vi "Begin.vi"(11 "Image Size":T1=enum."160x120") -> (0 "error out":errorcluster)   [LabVIEW 2013]
doc: "Called before other user functions, this VI is expected to open initial I/O refnums, load in file data, and do all program initialization. Notice that the <B>error out</B> terminal is simply used for data flow. Wiring it to other structures or subVIs ensures that this VI runs first."
uses:
  <vilib>/Rock Robotics/WPI/Camera/WPI_CameraImageSize.ctl
  <vilib>/Rock Robotics/WPI/Camera/WPI_CameraWhite Balance Values.ctl
  <vilib>/Rock Robotics/WPI/Camera/WPI_CameraExposure Values.ctl
  <vilib>/Rock Robotics/WPI/Camera/WPI_CameraFrameRate.ctl
  <vilib>/Rock Robotics/WPI/DriverStation/WPI_DriverStationRobotMode2.ctl
  <vilib>/Rock Robotics/WPI/Joystick/WPI_JoystickDeviceEnum.ctl
  <vilib>/Rock Robotics/SystemInterfaces/DIO/FPGA_DIOPWMChannel.ctl
  <vilib>/Rock Robotics/SystemInterfaces/DIO/FPGA_DIOChannel.ctl
  <vilib>/Rock Robotics/WPI/Solenoid/WPI_SolenoidChannel.ctl
  <vilib>/Rock Robotics/SystemInterfaces/DIO/FPGA_DIORelayChannel.ctl
  <vilib>/Rock Robotics/WPI/SafetyOutput/WPI_SafetyOutputConfigMenu.ctl
  <vilib>/Rock Robotics/SystemInterfaces/Typedef/FPGA_TypedefSolenoidModule.ctl
  <vilib>/Rock Robotics/WPI/Encoder/WPI_EncoderType.ctl
  <vilib>/Rock Robotics/WPI/Relay/WPI_RelayValue.ctl
  <vilib>/Rock Robotics/SystemInterfaces/Typedef/FPGA_TypedefDigitalModule.ctl
  Robot Global Data.vi
  <vilib>/Rock Robotics/WPI/MotorControl/WPI_MotorControlOpen Talon.vi
  <vilib>/Rock Robotics/WPI/Counter/WPI_CounterDigitalInputToDigitalSource.vi
  <vilib>/Rock Robotics/WPI/RobotDrive/WPI_RobotDriveOpen2MotorWithTalon.vi
  <vilib>/Rock Robotics/WPI/Solenoid/WPI_SolenoidOpenDouble.vi
  <vilib>/Rock Robotics/WPI/Compressor/WPI_CompressorGetSetRefNum.vi
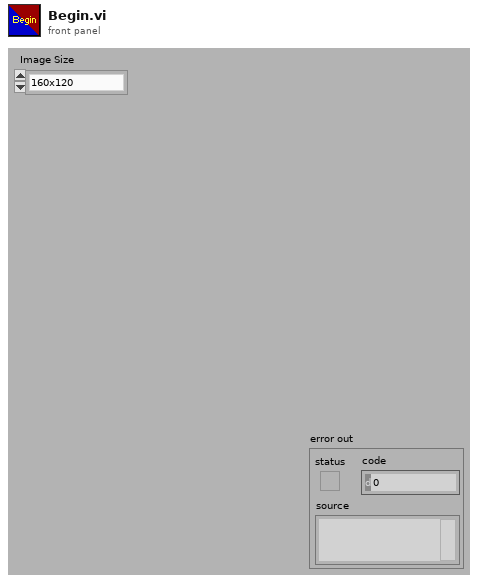
[diagram p1: front panel]
types:
  T1 = typedef "WPI_CameraImageSize.ctl" = enum16{"640x480", "320x240", "160x120"}
  T2 = typedef "FPGA_DIOPWMChannel.ctl" = enum8{"PWM 1", "PWM 2", "PWM 3", "PWM 4", "PWM 5", "PWM 6", "PWM 7", "PWM 8", "PWM 9", "PWM 10", "Invalid"}
  T3 = typedef "FPGA_TypedefDigitalModule.ctl" = enum16{"Digital Module 1", "Digital Module 2"}
  T4 = typedef "WPI_RelayValue.ctl" = enum16{"Off", "On", "Forward", "Reverse"}
  T5 = typedef "FPGA_DIORelayChannel.ctl" = enum8{"Relay 1", "Relay 2", "Relay 3", "Relay 4", "Relay 5", "Relay 6", "Relay 7", "Relay 8", "Invalid"}
  T6 = typedef "WPI_EncoderType.ctl" = enum16{"1x", "2x", "4x"}
  T7 = typedef "FPGA_DIOChannel.ctl" = enum8{"DIO 1", "DIO 2", "DIO 3", "DIO 4", "DIO 5", "DIO 6", "DIO 7", "DIO 8", "DIO 9", "DIO 10", "DIO 11", "DIO 12", "DIO 13", "DIO 14", "Invalid"}
  T8 = typedef "FPGA_TypedefSolenoidModule.ctl" = enum16{"Solenoid Module 1", "Solenoid Module 2"}
  T9 = typedef "WPI_SafetyOutputConfigMenu.ctl" = enum16{"Enable", "Disable"}
  T10 = typedef "WPI_SolenoidChannel.ctl" = enum8{"Solenoid 1", "Solenoid 2", "Solenoid 3", "Solenoid 4", "Solenoid 5", "Solenoid 6", "Solenoid 7", "Solenoid 8", "Invalid"}
  T11 = typedef "WPI_JoystickDeviceEnum.ctl" = enum16{"USB 1", "USB 2", "USB 3", "USB 4", "Kinect 1", "Kinect 2"}
  T12 = typedef "WPI_DriverStationRobotMode2.ctl" = enum16{"Autonomous Disabled", "Autonomous Enabled", "Teleop Disabled", "Teleop Enabled", "Timeout", "Finish", "Test Disabled", "Test Enabled"}
  T13 = typedef "WPI_CameraFrameRate.ctl" = u32
  T14 = typedef "WPI_CameraExposure Values.ctl" = enum16{"Auto", "Flicker-free 50 Hz", "Flicker-free 60 Hz", "Hold current"}
  T15 = typedef "WPI_CameraWhite Balance Values.ctl" = enum16{"Auto", "Fixed indoor", "Fixed outdoor 1", "Fixed outdoor 2", "Fixed fluorescent 1", "Fixed fluorescent 2", "Hold current"}
  T16 = typedef "WPI_JoystickDevRef.ctl" = cluster{"Device":T11}
  T17 = typedef "WPI_RobotDriveDevRef.ctl" = cluster{"DevStatus":errorcluster, "Motors[]":T18[], "Square Inputs":bool, "Max Output":dbl, "Isochronous":bool}
  T18 = typedef "WPI_MotorControlDeviceRef.ctl" = cluster{"DeviceStatus":errorcluster, "Type":enum16{"PWM", "CAN"}, "PWM":cluster{"Digital Module":T3, "PWM Channel":T2, "DeadBand":T19}, "CAN":cluster{"Device Number":u8, "Control Mode":T20, "Semaphore":T21, "Max Vout":dbl}, "Invert":bool, "TransformRef":T22, "InvTransformRef":T22}
  T19 = typedef "WPI_PWMDeadband.ctl" = cluster{"Name":string, "maxPositivePwm":i32, "minPositivePwm":i32, "centerPwm":i32, "maxNegativePwm":i32, "minNegativePwm":i32, "angularRange":u16}
  T20 = typedef "WPI_CANJaguar_ControlMode.ctl" = enum8{"Percent VBus", "Current", "Speed", "Position", "Voltage"}
  T21 = typedef "Semaphore RefNum" = refnum<k1>
  T22 = typedef "WPI_PWMTransform_ConPane.ctl" = refnum<vi>
  T23 = typedef "WPI_CameraDevRef.ctl" = cluster{"Camera Address":string, "CameraStatus":errorcluster, "Acquire Image Notifier":refnum<notifier>}
  T24 = typedef "WPI_DigitalInputDevRef.ctl" = cluster{"DevStatus":errorcluster, "DIO Channel":T7, "Digital Module":T3}
  T25 = typedef "WPI_CompressorDevRef.ctl" = cluster{"DevStatus":errorcluster, "DigitalInputDevRef":T24, "RelayDevRef":T26}
  T26 = typedef "WPI_RelayDevRef.ctl" = cluster{"DevStatus":errorcluster, "Relay Channel":T5, "Digital Module":T3, "Relay Direction":T27}
  T27 = typedef "WPI_RelayDirection.ctl" = enum16{"Both directions", "Forward only", "Reverse only"}
  T28 = typedef "FPGA_CounterEncoderSourceConvertionLVSourceType.ctl" = cluster{"DevStatus":errorcluster, "AnalogTriggerMode?":bool, "DigitalMode":cluster{"Digital Module":T3, "DIO Channel":T29}, "AnalogTriggerMode":cluster{"AnalogTriggerIndex":T30, "OutputType":T31}}
  T29 = typedef "FPGA_DIODigitalSourceChannel.ctl" = enum8{"DIO 1", "DIO 2", "DIO 3", "DIO 4", "DIO 5", "DIO 6", "DIO 7", "DIO 8", "DIO 9", "DIO 10", "DIO 11", "DIO 12", "DIO 13", "DIO 14", "Disabled"}
  T30 = typedef "FPGA_AnalogTriggerIndex.ctl" = enum8{"Trig 0", "Trig 1", "Trig 2", "Trig 3", "Trig 4", "Trig 5", "Trig 6", "Trig 7", "Invalid"}
  T31 = typedef "FPGA_AnalogTriggerOutType.ctl" = enum16{"InWindow", "TriggerState", "Rising", "Falling"}
  T32 = typedef "WPI_EncoderDevRef.ctl" = cluster{"DevStatus":errorcluster, "EncoderIndex":T33, "CounterIndex":T34, "DistancePerCount":dbl, "Decoding Type":T6}
  T33 = typedef "FPGA_EncoderIdx.ctl" = enum8{"Enc 0", "Enc 1", "Enc 2", "Enc 3", "Invalid"}
  T34 = typedef "FPGA_CounterCtrSystemIndex.ctl" = enum8{"Ctr 0", "Ctr 1", "Ctr 2", "Ctr 3", "Ctr 4", "Ctr 5", "Ctr 6", "Ctr 7", "Invalid"}
  T35 = typedef "WPI_SolenoidDevRef.ctl" = cluster{"DevStatus":errorcluster, "Solenoid Module":T8, "Forward Solenoid Channel":T10, "Reverse Solenoid Channel":T10}
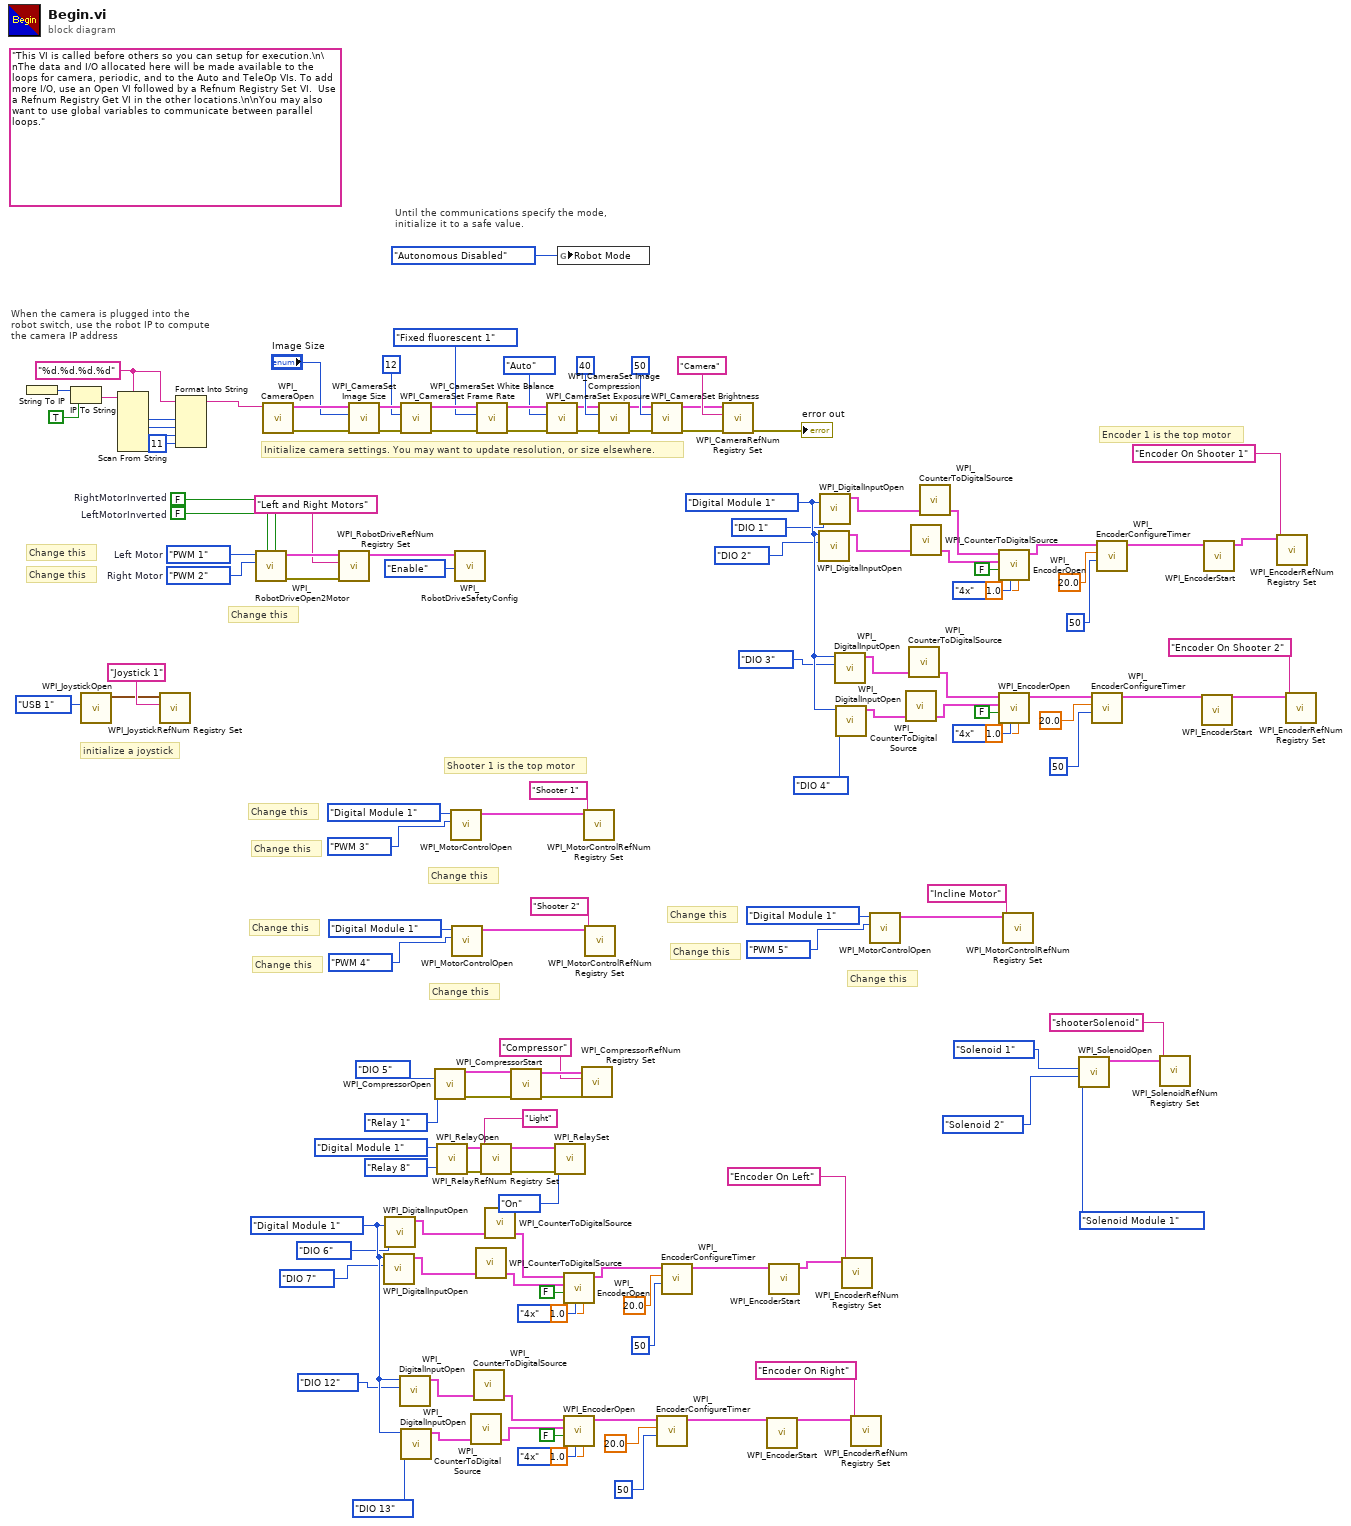
[diagram p0: block diagram]
diagram:
  w43 = FPGA_TypedefDigitalModule."Digital Module 1" ("Digital Module (Module 1)")
  w49 = FPGA_DIOPWMChannel."PWM 2"  # Right Motor
  w50 = FPGA_DIOPWMChannel."PWM 1"  # Left Motor
  w54 = FALSE  # LeftMotorInverted
  w55 = FALSE  # RightMotorInverted
  w96 = FPGA_TypedefDigitalModule."Digital Module 1" ("Digital Module (Module 1)")
  w111 = "%d.%d.%d.%d" ("format string")
  (unwired) "This VI is called before others so you can setup for execution.\n\nThe data and I/O allocated here will be made available to the loops for camera, periodic, and to the Auto and TeleOp VIs. To add more I/O, use an Open VI followed by a Refnum Registry Set VI.  Use a Refnum Registry Get VI in the other locations.\n\nYou may also want to use global variables to communicate between parallel loops."
  # "Change this"
  # "Change this"
  # "Change this"
  # "Shooter 1 is the top motor"
  # "Encoder 1 is the top motor"
  # "Change this"
  # "Change this"
  # "Change this"
  # "Change this"
  # "Change this"
  # "Change this"
  # "Change this"
  # "Change this"
  # "Change this"
  # "initialize a joystick"
  # "Until the communications specify the mode,\ninitialize it to a safe value."
  # "When the camera is plugged into the\nrobot switch, use the robot IP to compute\nthe camera IP address"
  # "Initialize camera settings. You may want to update resolution, or size elsewhere."
  n1 = String To IP() -> (0:w117:u32)  [unwired: 1 in]
  n2 = IP To String(1:TRUE ("dot notation? (F)"), 2:w117) -> (0:w115:string)
  n3 = call <vilib>:"WPI_JoystickOpen.vi"("JoystickDevice"=WPI_JoystickDeviceEnum."USB 1") -> ("JoystickDevRef"=w107:T16)  [unwired: 10 in]
  n4 = Scan From String(format string=w111, input string=w115) -> (output 1=w114:i32, output 2=w113:i32, output 3=w112:i32)  [unwired: 7 in, 3 out]
  n5 = call <vilib>:"WPI_JoystickRefNum Registry Set.vi"("refnum name"="Joystick 1", "JoystickDevRef"=w107) -> ()  [unwired: 8 in, 2 out]
  n6 = Format Into String(format string=w111, w114, w113, w112, 11 ("input 4")) -> (resulting string=w109:string)  [unwired: 2 in, 1 out]
  n7 = call-poly <vilib>:"WPI_RobotDriveOpen2Motor.vi"("Right Motor Inverted"=w55, "Left Motor Inverted"=w54, "Right Motor"=w49, "Left Motor"=w50) -> ("error out"=w51:errorcluster, "RobotDriveDevRef"=w53:T17)  [unwired: 1 in, 5 out]
  n8 = call <vilib>:"WPI_CameraOpen.vi"("Camera Address"=w109) -> ("error out"=w129:errorcluster, "CameraDevRef"=w130:T23)  [unwired: 1 in, 8 out]
  n9 = call <vilib>:"WPI_RobotDriveRefNum Registry Set.vi"("error in (no error)"=w51, "refnum name"="Left and Right Motors", "RobotDriveDevRef"=w53) -> ("RobotDriveDevRef"=w48:T17)  [unwired: 8 out]
  n10 = call <vilib>:"WPI_CameraSet Image Size.vi"("error in (no error)"=w129, "Image Size"="Image Size", "CameraDevRef"=w130) -> ("error out"=w128:errorcluster, "CameraDevRef Out"=w131:T23)  [unwired: 7 out]
  n11 = call <vilib>:"WPI_DigitalInputOpen.vi"("DIO Channel"=FPGA_DIOChannel."DIO 7", "Digital Module (Module 1)"=w43) -> ("DigitalInputDevRef"=w36:T24)  [unwired: 8 in, 1 out]
  n12 = call <vilib>:"WPI_DigitalInputOpen.vi"("DIO Channel"=FPGA_DIOChannel."DIO 6", "Digital Module (Module 1)"=w43) -> ("DigitalInputDevRef"=w35:T24)  [unwired: 8 in, 1 out]
  n13 = call <vilib>:"WPI_DigitalInputOpen.vi"("DIO Channel"=FPGA_DIOChannel."DIO 12", "Digital Module (Module 1)"=w43) -> ("DigitalInputDevRef"=w37:T24)  [unwired: 8 in, 1 out]
  n14 = call <vilib>:"WPI_CameraSet Frame Rate.vi"("error in (no error)"=w128, "Frame Rate (fps)"=T13 12, "CameraDevRef"=w131) -> ("error out"=w127:errorcluster, "CameraDevRef Out"=w133:T23)  [unwired: 7 out]
  n15 = call <vilib>:"WPI_DigitalInputOpen.vi"("DIO Channel"=FPGA_DIOChannel."DIO 13", "Digital Module (Module 1)"=w43) -> ("DigitalInputDevRef"=w38:T24)  [unwired: 8 in, 1 out]
  n16 = call <vilib>:"WPI_CompressorOpen.vi"("Pressure Switch DIO Channel"=FPGA_DIOChannel."DIO 5", "Relay Channel"=FPGA_DIORelayChannel."Relay 1") -> ("CompressorDevRef"=w63:T25, "error out"=w61:errorcluster)  [unwired: 12 in]
  n17 = call <vilib>:"WPI_RelayOpen.vi"("Relay Channel"=FPGA_DIORelayChannel."Relay 8", "Digital Module (Module 1)"=FPGA_TypedefDigitalModule."Digital Module 1") -> ("error out"=w12:errorcluster, "RelayDevRef"=w11:T26)  [unwired: 8 in]
  n18 = call-poly <vilib>:"WPI_MotorControlOpen.vi"("PWM Channel"=FPGA_DIOPWMChannel."PWM 3", "Digital Module (Module 1)"=FPGA_TypedefDigitalModule."Digital Module 1") -> ("MotorControlDeviceRef"=w102:T18)  [unwired: 8 in, 1 out]
  n19 = call-poly <vilib>:"WPI_MotorControlOpen.vi"("PWM Channel"=FPGA_DIOPWMChannel."PWM 4", "Digital Module (Module 1)"=FPGA_TypedefDigitalModule."Digital Module 1") -> ("MotorControlDeviceRef"=w98:T18)  [unwired: 8 in, 1 out]
  n20 = call <vilib>:"WPI_RobotDriveSafetyConfig.vi"("mode"=WPI_SafetyOutputConfigMenu."Enable", "RobotDriveDevRef"=w48) -> ()  [unwired: 8 in, 2 out]
  n21 = call-poly <vilib>:"WPI_CounterToDigitalSource.vi"("DigitalInputDevRef"=w38) -> ("Digital Source"=w31:T28)  [unwired: 6 in]
  n22 = call-poly <vilib>:"WPI_CounterToDigitalSource.vi"("DigitalInputDevRef"=w37) -> ("Digital Source"=w32:T28)  [unwired: 6 in]
  n23 = call-poly <vilib>:"WPI_CounterToDigitalSource.vi"("DigitalInputDevRef"=w36) -> ("Digital Source"=w33:T28)  [unwired: 6 in]
  n24 = call <vilib>:"WPI_CameraSet White Balance.vi"("error in (no error)"=w127, "White Balance"=WPI_CameraWhite_Balance_Values."Fixed fluorescent 1", "CameraDevRef"=w133) -> ("error out"=w126:errorcluster, "CameraDevRef Out"=w132:T23)  [unwired: 7 out]
  n25 = call <vilib>:"WPI_RelayRefNum Registry Set.vi"("error in (no error)"=w12, "refnum name"="Light", "RelayDevRef"=w11) -> ("error out"=w7:errorcluster, "RelayDevRef"=w6:T26)  [unwired: 7 in]
  n26 = call-poly <vilib>:"WPI_CounterToDigitalSource.vi"("DigitalInputDevRef"=w35) -> ("Digital Source"=w34:T28)  [unwired: 6 in]
  n27 = call <vilib>:"WPI_CompressorStart.vi"("error in (no error)"=w61, "CompressorDevRef"=w63) -> ("error out"=w60:errorcluster, "CompressorDevRef"=w62:T25)  [unwired: 8 in]
  n28 = call <vilib>:"WPI_CameraSet Exposure.vi"("error in (no error)"=w126, "Exposure"=WPI_CameraExposure_Values."Auto", "CameraDevRef"=w132) -> ("error out"=w125:errorcluster, "CameraDevRef Out"=w135:T23)  [unwired: 7 out]
  n29 = call <vilib>:"WPI_RelaySet.vi"("error in (no error)"=w7, "RelayValue"=WPI_RelayValue."On", "RelayDevRef"=w6) -> ()  [unwired: 7 in, 2 out]
  n30 = global write "Robot Global Data.vi" "Robot Mode"(WPI_DriverStationRobotMode2."Autonomous Disabled" ("Robot Mode")) -> ()
  n31 = call <vilib>:"WPI_EncoderOpen.vi"("DistancePerCount"=1.0, "Decoding Type"=WPI_EncoderType."4x", "Invert Direction (False)"=FALSE, "BSource"=w33, "ASource"=w34) -> ("EncoderDevRef"=w30:T32)  [unwired: 5 in, 1 out]
  n32 = call <vilib>:"WPI_EncoderOpen.vi"("DistancePerCount"=1.0, "Decoding Type"=WPI_EncoderType."4x", "Invert Direction (False)"=FALSE, "BSource"=w31, "ASource"=w32) -> ("EncoderDevRef"=w29:T32)  [unwired: 5 in, 1 out]
  n33 = call <vilib>:"WPI_CompressorRefNum Registry Set.vi"("error in (no error)"=w60, "refnum name"="Compressor", "CompressorDevRef"=w62) -> ()  [unwired: 7 in, 2 out]
  n34 = call <vilib>:"WPI_MotorControlRefNum Registry Set.vi"("refnum name"="Shooter 1", "MotorControlDevRef"=w102) -> ()  [unwired: 8 in, 2 out]
  n35 = call <vilib>:"WPI_MotorControlRefNum Registry Set.vi"("refnum name"="Shooter 2", "MotorControlDevRef"=w98) -> ()  [unwired: 8 in, 2 out]
  n36 = call <vilib>:"WPI_CameraSet Image Compression.vi"("error in (no error)"=w125, "Compression"=40, "CameraDevRef"=w135) -> ("error out"=w124:errorcluster, "CameraDevRef Out"=w134:T23)  [unwired: 7 out]
  n37 = call <vilib>:"WPI_CameraSet Brightness.vi"("error in (no error)"=w124, "Brightness"=50, "CameraDevRef"=w134) -> ("error out"=w122:errorcluster, "CameraDevRef Out"=w123:T23)  [unwired: 7 out]
  n38 = call <vilib>:"WPI_EncoderConfigureTimer.vi"("Number Samples to Average"=u8 50, "Minimum Rate"=20.0, "EncoderDevRef"=w29) -> ("EncoderDevRef"=w27:T32)  [unwired: 7 in, 1 out]
  n39 = call <vilib>:"WPI_EncoderConfigureTimer.vi"("Number Samples to Average"=u8 50, "Minimum Rate"=20.0, "EncoderDevRef"=w30) -> ("EncoderDevRef"=w28:T32)  [unwired: 7 in, 1 out]
  n40 = call <vilib>:"WPI_CameraRefNum Registry Set.vi"("error in (no error)"=w122, "refnum name"="Camera", "CameraDevRef"=w123) -> ("error out"=→"error out":errorcluster)  [unwired: 8 out]
  n41 = call <vilib>:"WPI_EncoderStart.vi"("EncoderDevRef"=w27) -> ("EncoderDevRef"=w26:T32)  [unwired: 9 in, 1 out]
  n42 = call <vilib>:"WPI_EncoderStart.vi"("EncoderDevRef"=w28) -> ("EncoderDevRef"=w25:T32)  [unwired: 9 in, 1 out]
  n43 = call <vilib>:"WPI_DigitalInputOpen.vi"("DIO Channel"=FPGA_DIOChannel."DIO 2", "Digital Module (Module 1)"=w96) -> ("DigitalInputDevRef"=w89:T24)  [unwired: 8 in, 1 out]
  n44 = call <vilib>:"WPI_DigitalInputOpen.vi"("DIO Channel"=FPGA_DIOChannel."DIO 1", "Digital Module (Module 1)"=w96) -> ("DigitalInputDevRef"=w88:T24)  [unwired: 8 in, 1 out]
  n45 = call <vilib>:"WPI_DigitalInputOpen.vi"("DIO Channel"=FPGA_DIOChannel."DIO 3", "Digital Module (Module 1)"=w96) -> ("DigitalInputDevRef"=w90:T24)  [unwired: 8 in, 1 out]
  n46 = call <vilib>:"WPI_DigitalInputOpen.vi"("DIO Channel"=FPGA_DIOChannel."DIO 4", "Digital Module (Module 1)"=w96) -> ("DigitalInputDevRef"=w91:T24)  [unwired: 8 in, 1 out]
  n47 = call <vilib>:"WPI_EncoderRefNum Registry Set.vi"("refnum name"="Encoder On Left", "EncoderDevRef"=w25) -> ()  [unwired: 8 in, 2 out]
  n48 = call <vilib>:"WPI_EncoderRefNum Registry Set.vi"("refnum name"="Encoder On Right", "EncoderDevRef"=w26) -> ()  [unwired: 8 in, 2 out]
  n49 = call-poly <vilib>:"WPI_MotorControlOpen.vi"("PWM Channel"=FPGA_DIOPWMChannel."PWM 5", "Digital Module (Module 1)"=FPGA_TypedefDigitalModule."Digital Module 1") -> ("MotorControlDeviceRef"=w2:T18)  [unwired: 8 in, 1 out]
  n50 = call-poly <vilib>:"WPI_CounterToDigitalSource.vi"("DigitalInputDevRef"=w91) -> ("Digital Source"=w84:T28)  [unwired: 6 in]
  n51 = call-poly <vilib>:"WPI_CounterToDigitalSource.vi"("DigitalInputDevRef"=w90) -> ("Digital Source"=w85:T28)  [unwired: 6 in]
  n52 = call-poly <vilib>:"WPI_CounterToDigitalSource.vi"("DigitalInputDevRef"=w89) -> ("Digital Source"=w86:T28)  [unwired: 6 in]
  n53 = call-poly <vilib>:"WPI_CounterToDigitalSource.vi"("DigitalInputDevRef"=w88) -> ("Digital Source"=w87:T28)  [unwired: 6 in]
  n54 = call <vilib>:"WPI_EncoderOpen.vi"("DistancePerCount"=1.0, "Decoding Type"=WPI_EncoderType."4x", "Invert Direction (False)"=FALSE, "BSource"=w86, "ASource"=w87) -> ("EncoderDevRef"=w83:T32)  [unwired: 5 in, 1 out]
  n55 = call <vilib>:"WPI_EncoderOpen.vi"("DistancePerCount"=1.0, "Decoding Type"=WPI_EncoderType."4x", "Invert Direction (False)"=FALSE, "BSource"=w84, "ASource"=w85) -> ("EncoderDevRef"=w82:T32)  [unwired: 5 in, 1 out]
  n56 = call <vilib>:"WPI_MotorControlRefNum Registry Set.vi"("refnum name"="Incline Motor", "MotorControlDevRef"=w2) -> ()  [unwired: 8 in, 2 out]
  n57 = call-poly <vilib>:"WPI_SolenoidOpen.vi"("Reverse Solenoid Channel"=WPI_SolenoidChannel."Solenoid 2", "Forward Solenoid Channel"=WPI_SolenoidChannel."Solenoid 1", "Solenoid Module (Module 1)"=FPGA_TypedefSolenoidModule."Solenoid Module 1") -> ("SolenoidDevRef"=w64:T35)  [unwired: 7 in, 1 out]
  n58 = call <vilib>:"WPI_EncoderConfigureTimer.vi"("Number Samples to Average"=u8 50, "Minimum Rate"=20.0, "EncoderDevRef"=w82) -> ("EncoderDevRef"=w80:T32)  [unwired: 7 in, 1 out]
  n59 = call <vilib>:"WPI_EncoderConfigureTimer.vi"("Number Samples to Average"=u8 50, "Minimum Rate"=20.0, "EncoderDevRef"=w83) -> ("EncoderDevRef"=w81:T32)  [unwired: 7 in, 1 out]
  n60 = call <vilib>:"WPI_SolenoidRefNum Registry Set.vi"("refnum name"="shooterSolenoid", "SolenoidDevRef"=w64) -> ()  [unwired: 8 in, 2 out]
  n61 = call <vilib>:"WPI_EncoderStart.vi"("EncoderDevRef"=w80) -> ("EncoderDevRef"=w79:T32)  [unwired: 9 in, 1 out]
  n62 = call <vilib>:"WPI_EncoderStart.vi"("EncoderDevRef"=w81) -> ("EncoderDevRef"=w78:T32)  [unwired: 9 in, 1 out]
  n63 = call <vilib>:"WPI_EncoderRefNum Registry Set.vi"("refnum name"="Encoder On Shooter 1", "EncoderDevRef"=w78) -> ()  [unwired: 8 in, 2 out]
  n64 = call <vilib>:"WPI_EncoderRefNum Registry Set.vi"("refnum name"="Encoder On Shooter 2", "EncoderDevRef"=w79) -> ()  [unwired: 8 in, 2 out]
